vi "simulate_database.vi"() -> ()   [LabVIEW 2011]
uses:
  <vilib>/addons/database/Connection.llb/DB Tools Open Connec (String).vi
  <vilib>/addons/database/NI_Database_API.lvlib
panel:
  out "deque error":errorcluster
  in  "stop 3":bool
  out "last received data":cluster{string, string, dbl, string, string}
  out "DB write error":errorcluster
  out "Number of \nreceived data":i32
  out "error in receiving data":errorcluster
  out "concatenated string":string
  in  "timestamp":string
  in  "stop 2":bool
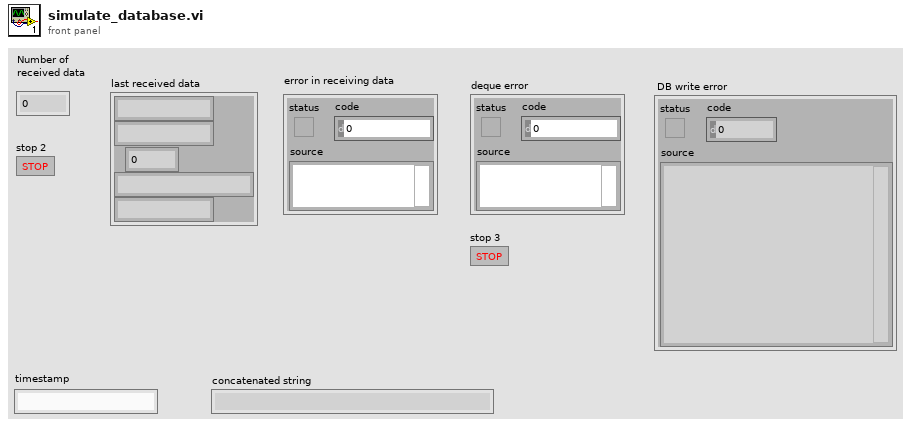
[diagram p1: front panel]
types:
  T1 = enum16{"Read", "Write", "ReadWrite", "BufferedRead", "BufferedReadWrite"}
  T2 = typedef "NI_Database_API.lvlib/Conn ObjectReference.ctl" = refnum<k1>
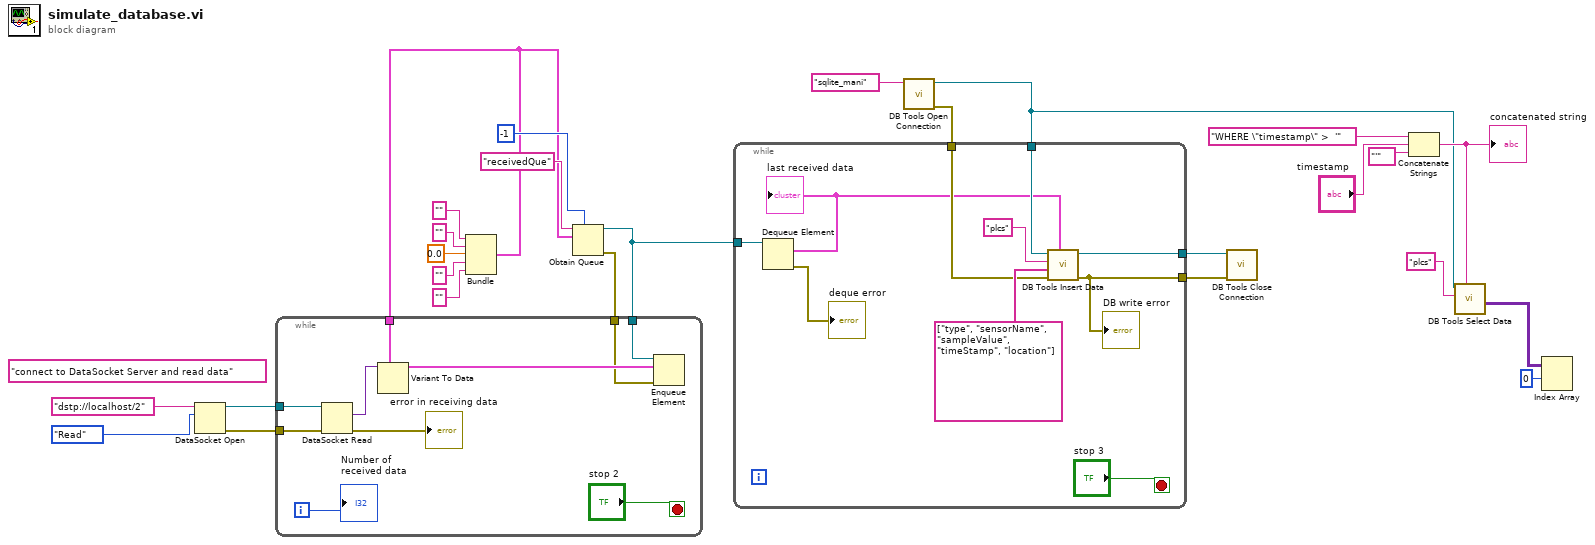
[diagram p0: block diagram]
diagram:
  (unwired) "connect to DataSocket Server and read data"
  n1 = DataSocket Open(10:T1."Read" ("mode"), 11:"dstp://localhost/2" ("URL 3")) -> (0:w18:errorcluster, 3:w17:refnum<k13>)  [unwired: 2 in]
  n2 = Bundle("", "", 0.0, "", "") -> (w3:cluster{string, string, dbl, string, string})  [unwired: 1 in]
  n3 = Obtain Queue(max queue size (-1, unlimited)=-1, name (unnamed)="receivedQue", element data type=w3) -> (queue out=w8:refnum<queue>, error out=w9:errorcluster)  [unwired: 2 in, 1 out]
  n4 = while {
    tunnel: w18 -> [w33]
    tunnel: w17 -> [w32]
    tunnel: w3 -> [w30]
    tunnel: w8 -> [w28]
    tunnel: w9 -> [w27]
    i -> [w35]
    stop <- "stop 2" stop-if-true
    n5 = DataSocket Read(8:w33, 11:w32) -> (0:→"error in receiving data":errorcluster, 2:w31:variant)  [unwired: 3 in, 5 out]
    n6 = Variant To Data(type=w30, Variant=w31) -> (data=w29:cluster{string, string, dbl, string, string})  [unwired: 1 in, 1 out]
    n7 = Enqueue Element(queue=w28, element=w29, error in (no error)=w27) -> ()  [unwired: 1 in, 3 out]
    "Number of \nreceived data" <- w35
  }
  n8 = call-poly <vilib>:"DB Tools Open Connection.vi"("connection information"="sqlite_mani") -> ("error out"=w7:errorcluster, "connection reference"=w4:T2)  [unwired: 7 in]
  n9 = while {
    tunnel: w8 -> [w42]
    tunnel: w7 -> [w41]
    tunnel: w4 -> [w40]
    tunnel: [w39] -> w6
    tunnel: [w38] -> w5
    stop <- "stop 3" stop-if-true
    n10 = Dequeue Element(queue=w42) -> (element=w37:cluster{string, string, dbl, string, string}, error out=→"deque error":errorcluster)  [unwired: 2 in, 2 out]
    "last received data" <- w37
    n11 = call <vilib>:"DB Tools Insert Data.vi"("data"=w37, "error in (no error)"=w41, "columns"=string[] ["type", "sensorName", "sampleValue", "timeStamp", "location"], "table"="plcs", "connection reference"=w40) -> ("error out"=w38:errorcluster, "connection reference out"=w39:T2)  [unwired: 5 in]
    "DB write error" <- w38
  }
  n12 = call <vilib>:"DB Tools Close Connection.vi"("error in (no error)"=w5, "connection reference"=w6) -> ()  [unwired: 5 in, 1 out]
  n13 = Concatenate Strings("WHERE \"timestamp\" >  '", "timestamp", "'") -> (w21:string)
  "concatenated string" <- w21
  n14 = call <vilib>:"DB Tools Select Data.vi"("condition"=w21, "table"="plcs", "connection reference"=w4) -> ("data"=w2:variant[][])  [unwired: 3 in, 2 out]
  n15 = Index Array(array=w2, index (row)=0) -> ()  [unwired: 1 in, 1 out]
